vi "SaveCycleSweep.vi"(5 "Area":dbl=1.0, 6 "JunctionName":string, 7 "SideLength":dbl=1.0, 8 "UiDefinition 2":T3, 9 "InfoCluster":T1, 10 "appended array":dbl[][](array[numeric])) -> (0 "error out":errorcluster)   [LabVIEW 2020]
uses:
  Keithley_Subs/CapacitanceInfos.ctl
  Keithley_Subs/CapacitanceRecord.ctl
  UIReferences.ctl
  D:/LabviewDXFViewer/LabviewDXFViewer/bin/Release/LabviewDXFViewer.exe
  LabviewDXFViewer/bin/Release/LabviewDXFViewer.exe
  <vilib>/httpClient/POSTBuffer.vi
  <vilib>/httpClient/LabVIEWHTTPClient.lvlib
panel:
  in  "Cluster 3":T4
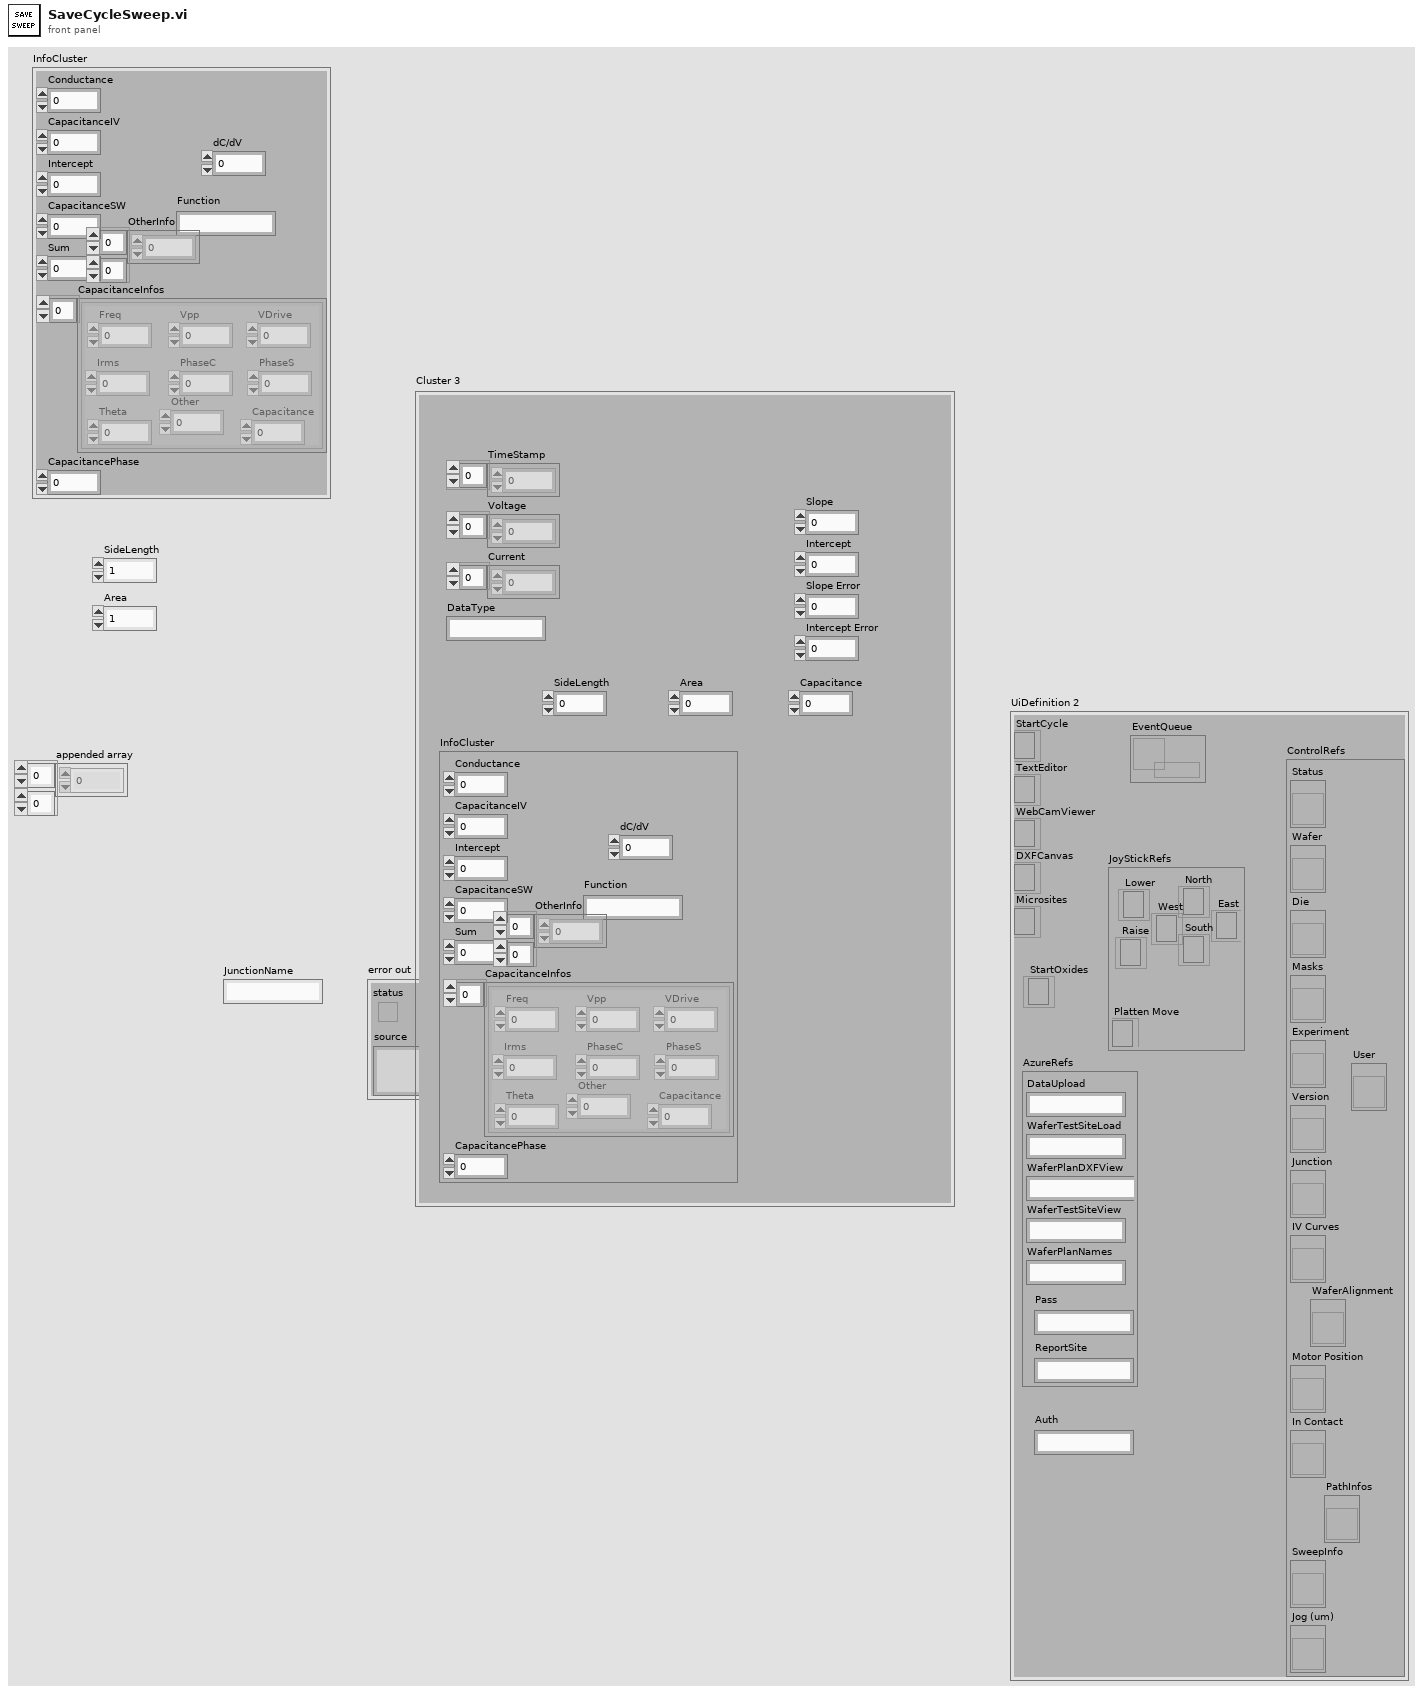
[diagram p1: front panel]
types:
  T1 = typedef "CapacitanceInfos.ctl" = cluster{"Conductance":dbl, "CapacitanceIV":dbl, "Intercept":dbl, "CapacitanceSW":dbl, "Sum":dbl, "CapacitanceInfos":T2[], "CapacitancePhase":dbl, "dC/dV":dbl, "Function":string, "OtherInfo":dbl[][]}
  T2 = typedef "CapacitanceRecord.ctl" = cluster{"Freq":dbl, "Vpp":dbl, "PhaseS":dbl, "Irms":dbl, "PhaseC":dbl, "Theta":dbl, "VDrive":dbl, "Capacitance":dbl, "Other":dbl}
  T3 = typedef "UIReferences.ctl" = cluster{"StartCycle":refnum<k24>, "TextEditor":refnum<k24>, "WebCamViewer":refnum<k24>, "DXFCanvas":refnum<k24>, "Microsites":refnum<k24>, "JoyStickRefs":cluster{"North":refnum<k24>, "Lower":refnum<k24>, "Raise":refnum<k24>, "Platten Move":refnum<k24>, "West":refnum<k24>, "East":refnum<k24>, "South":refnum<k24>}, "AzureRefs":cluster{"DataUpload":string, "WaferTestSiteLoad":string, "WaferPlanDXFView":string, "WaferTestSiteView":string, "WaferPlanNames":string, "Pass":string, "ReportSite":string}, "ControlRefs":cluster{"Status":refnum<vi>, "Wafer":refnum<vi>, "Die":refnum<vi>, "Masks":refnum<vi>, "Experiment":refnum<vi>, "Version":refnum<vi>, "Junction":refnum<vi>, "IV Curves":refnum<vi>, "Motor Position":refnum<vi>, "In Contact":refnum<vi>, "SweepInfo":refnum<vi>, "Jog (um)":refnum<vi>, "PathInfos":refnum<vi>, "User":refnum<vi>, "WaferAlignment":refnum<vi>}, "EventQueue":refnum<queue>, "StartOxides":refnum<k24>, "Auth":string}
  T4 = cluster{"Intercept Error":dbl, "Slope Error":dbl, "Intercept":dbl, "Slope":dbl, "DataType":string, "Current":dbl[], "Voltage":dbl[], "TimeStamp":dbl[], "Capacitance":dbl, "Area":dbl, "SideLength":dbl, "InfoCluster":T1}
  T5 = cluster{"Die":string, "Wafer":string, "Path":path, "url":string, "Experiment":string, "Version":string, "user":string}
  T6 = typedef "LabVIEWHTTPClient.lvlib/ClientHandle.ctl" = refnum<k1>
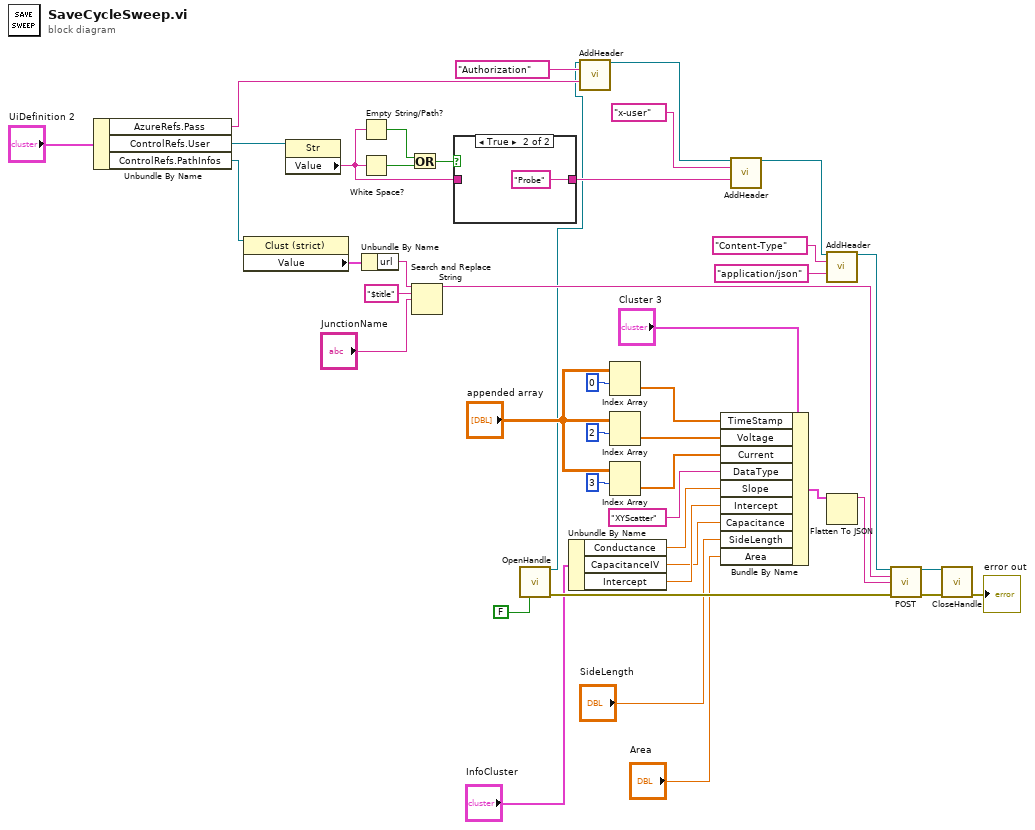
[diagram p0: block diagram]
diagram:
  n1 = Unbundle By Name("UiDefinition 2") -> ("AzureRefs.Pass"=w21:string, "ControlRefs.User"=w19:refnum<vi>, "ControlRefs.PathInfos"=w12:refnum<vi>)
  n2 = property class="Clust (strict)"(reference=w12) -> ("Value"=w11:T5)  [unwired: 1 in, 2 out]
  n3 = property class="Str"(reference=w19) -> ("Value"=w14:string)  [unwired: 1 in, 2 out]
  n4 = Empty String/Path?(string/path=w14) -> (empty?=w15:bool)
  n5 = White Space?(1:w14) -> (0:w18:bool)
  n6 = Unbundle By Name(w11) -> ("url"=w10:string)
  n7 = Or(x=w15, y=w18) -> (x .or. y?=w16:bool)
  n8 = Search and Replace String(input string=w10, search string="$title" ("string"), replace string="JunctionName") -> (result string=w28:string)  [unwired: 5 in, 3 out]
  n9 = case shown="True" w16 {
    tunnel: w14 -> [w45 _]
    tunnel: [w45 "Probe"] -> w17
    frame False {
    }
    frame True {
    }
  }
  n10 = call <vilib>:"OpenHandle.vi"("verify server(true)"=FALSE) -> ("client handle out"=w13:T6, "error out"=w43:errorcluster)  [unwired: 13 in]
  n11 = Unbundle By Name("InfoCluster") -> ("Conductance"=w9:dbl, "CapacitanceIV"=w7:dbl, "Intercept"=w8:dbl)
  n12 = call <vilib>:"AddHeader.vi"("client handle"=w13, "header"="Authorization", "value"=w21) -> ("client handle out"=w23:T6)  [unwired: 11 in, 1 out]
  n13 = Index Array(array="appended array", index (row)=0) -> (element=w35:dbl[])  [unwired: 1 in]
  n14 = Index Array(array="appended array", index (row)=2) -> (element=w38:dbl[])  [unwired: 1 in]
  n15 = Index Array(array="appended array", index (row)=3) -> (element=w39:dbl[])  [unwired: 1 in]
  n16 = Bundle By Name(cluster="Cluster 3", "TimeStamp"=w35, "Voltage"=w38, "Current"=w39, "DataType"="XYScatter", "Slope"=w9, "Intercept"=w8, "Capacitance"=w7, "SideLength"="SideLength", "Area"="Area") -> (w42:T4)
  n17 = call <vilib>:"AddHeader.vi"("client handle"=w23, "header"="x-user", "value"=w17) -> ("client handle out"=w2:T6)  [unwired: 11 in, 1 out]
  n18 = call <vilib>:"AddHeader.vi"("client handle"=w2, "header"="Content-Type", "value"="application/json") -> ("client handle out"=w1:T6)  [unwired: 11 in, 1 out]
  n19 = Flatten To JSON(anything=w42) -> (JSON string=w33:string)  [unwired: 2 in, 1 out]
  n20 = call-poly <vilib>:"POST.vi"("client handle"=w1, "url"=w28, "buffer"=w33, "error in (no error)"=w43) -> ("client handle out"=w31:T6, "error out"=w30:errorcluster)  [unwired: 8 in, 2 out]
  n21 = call <vilib>:"CloseHandle.vi"("client handle"=w31, "error in (no error)"=w30) -> ("error out"=→"error out":errorcluster)  [unwired: 13 in]
